vi "Change Recipe Label Control.vi"(8 "error in (no error)":errorcluster, 10 "Label":string, 11 "Recipe Window in":refnum<class "Recipe Window.lvclass">) -> (0 "error out":errorcluster, 3 "Recipe Window out":refnum<class "Recipe Window.lvclass">)   [LabVIEW 2021, in "Recipe.lvlib" / "Recipe Window.lvclass"]
uses:
  Recipe Window.lvclass
  Recipe Window.lvclass/Recipe Window.ctl
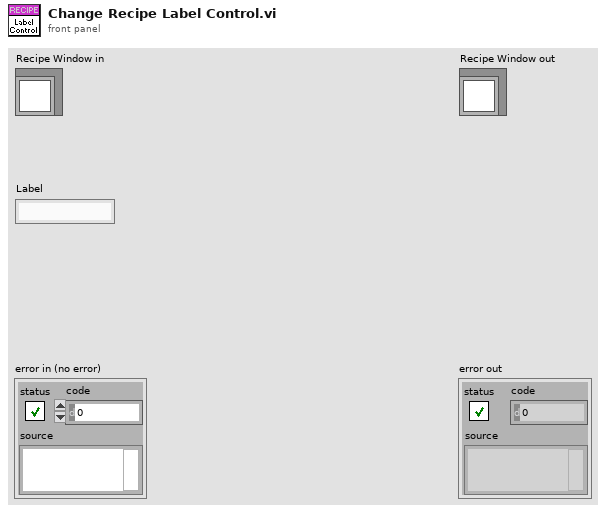
[diagram p1: front panel]
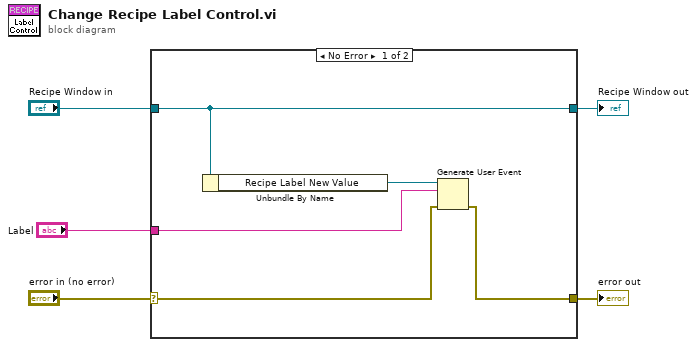
[diagram p0: block diagram]
diagram:
  n1 = case shown="No Error" "error in (no error)" {
    selector: "error in (no error)" -> [w9 w12]
    tunnel: [w8 w12] -> w4
    tunnel: [w10 w11] -> w2
    tunnel: "Recipe Window in" -> [w10 w11]
    tunnel: "Label" -> [w6 _]
    frame No Error {
      n2 = Unbundle By Name(w10) -> ("Recipe Label New Value"=w7:refnum<user-event>)
      n3 = Generate User Event(user event=w7, event data cluster=w6, error in=w9) -> (error out=w8:errorcluster)  [unwired: 1 in, 1 out]
    }
    frame Error {
    }
  }
  "error out" <- w4
  "Recipe Window out" <- w2
